vi "Get Image Date.vi"(8 "error in (no error)":errorcluster, 11 "Save Image in":refnum<class "Save Image.lvclass">) -> (0 "error out":errorcluster, 3 "Save Image out":refnum<class "Save Image.lvclass">)   [LabVIEW 2018, in "Save Image.lvclass"]
uses:
  Save Image.lvclass
  Save Image.lvclass/Save Image.ctl
  Simulated_Header/Simulated_Header.lvclass
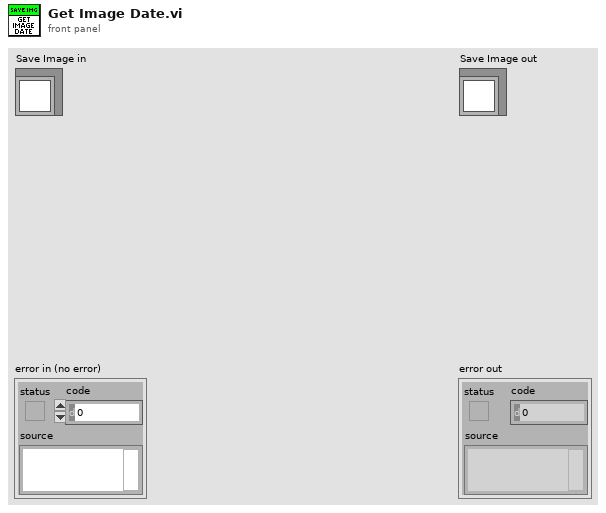
[diagram p1: front panel]
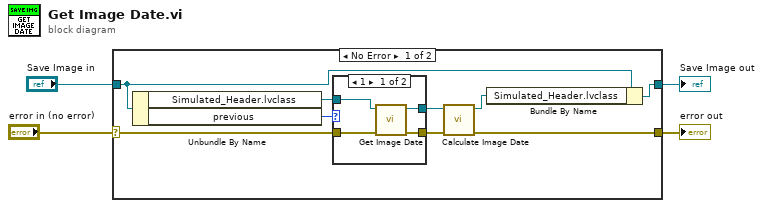
[diagram p0: block diagram]
diagram:
  n1 = case shown="No Error" "error in (no error)" {
    selector: "error in (no error)" -> [w13 w21]
    tunnel: [w5 w21] -> w3
    tunnel: [w10 w20] -> w1
    tunnel: "Save Image in" -> [w11 w20]
    frame No Error {
      n2 = Unbundle By Name(w11) -> ("Simulated_Header.lvclass"=w12:refnum<class "Simulated_Header.lvclass">, "previous"=w9:u16)
      n3 = case shown="1" w9 {
        tunnel: w13 -> [w17 w19]
        tunnel: w12 -> [w16 w18]
        tunnel: [w15 w18] -> w8
        tunnel: [w14 w19] -> w6
        frame 1 {
          n4 = call-dynamic "Get Image Date.vi"("error in (no error)"=w17, "Simulated_Header in"=w16) -> ("error out"=w14:errorcluster, "Simulated_Header out"=w15:refnum<class "Simulated_Header.lvclass">)  [unwired: 8 in]
        }
        frame 0, Default {
        }
      }
      n5 = call "Calculate Image Date.vi"("error in (no error)"=w6, "Simulated_Header in"=w8) -> ("error out"=w5:errorcluster, "Simulated_Header out"=w7:refnum<class "Simulated_Header.lvclass">)  [unwired: 8 in]
      n6 = Bundle By Name(cluster=w11, "Simulated_Header.lvclass"=w7) -> (w10:refnum<class "Save Image.lvclass">)
    }
    frame Error {
    }
  }
  "error out" <- w3
  "Save Image out" <- w1
